vi "GetLoopReference.vi"(8 "error in":errorcluster, 11 "Loop in":refnum<class "Loop.lvclass">) -> (0 "error out":errorcluster, 1 "reference out":refnum<vi>, 3 "Loop out":refnum<class "Loop.lvclass">)   [LabVIEW 2014, in "Loop.lvclass"]
uses:
  Loop.lvclass
  Generic/Generic.lvclass
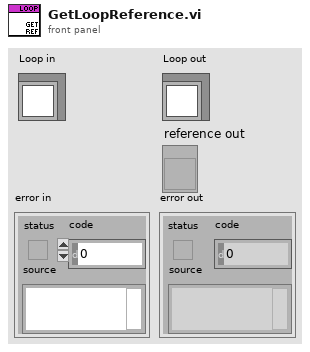
[diagram p1: front panel]
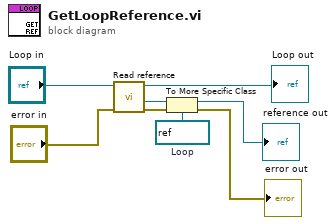
[diagram p0: block diagram]
diagram:
  w6 = refnum<vi> refnum  # Loop
  n1 = call "Read reference.vi"("error in"="error in", "GObject in"="Loop in") -> ("error out"=w7:errorcluster, "reference"=w8:refnum<vi>, "GObject out"=→"Loop out":refnum<class "Loop.lvclass">)  [unwired: 5 in]
  n2 = To More Specific Class(target class=w6, reference=w8, error in=w7) -> (specific class reference=→"reference out":refnum<vi>, error out=→"error out":errorcluster)
